vi "GetMeasCatalog.vi"(8 "error in (no error)":errorcluster, 10 "Channel":u32=1, 11 "NetA_AgNA in":refnum<class "NetA_AgNA.lvclass">) -> (0 "error out":errorcluster, 2 "Measurement Catalog":string, 3 "NetA_AgNA out":refnum<class "NetA_AgNA.lvclass">)   [LabVIEW 2014, in "NetA_AgNA.lvclass"]
doc: "Returns a list of measurements associated with the specified channel."
uses:
  NetA_AgNA.lvclass
  NetA_AgNA.lvclass/NetA_AgNA.ctl
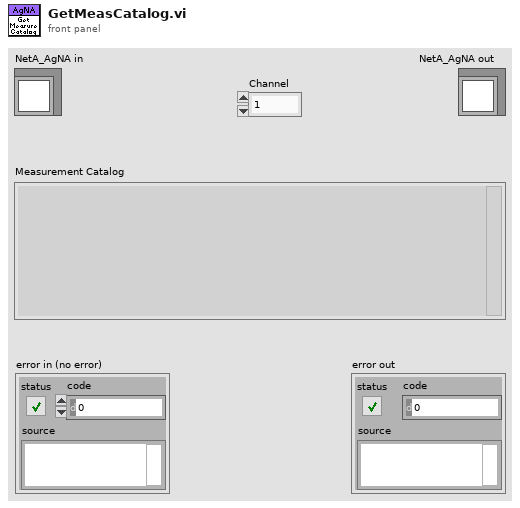
[diagram p1: front panel]
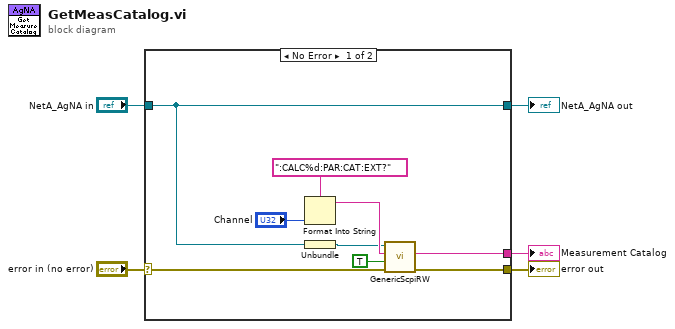
[diagram p0: block diagram]
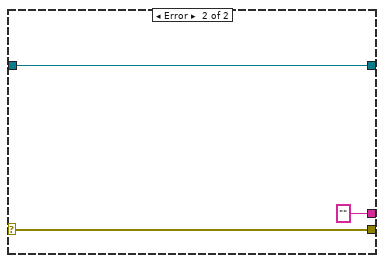
[diagram p2: hidden frame]
diagram:
  n1 = case shown="No Error" "error in (no error)" {
    selector: "error in (no error)" -> [w13 w16]
    tunnel: [w14 w16] -> w5
    tunnel: [w9 "" ("SCPI Response")] -> w3
    tunnel: "NetA_AgNA in" -> [w7 w17]
    tunnel: [w7 w17] -> w1
    frame No Error {
      n2 = Format Into String(format string=":CALC%d:PAR:CAT:EXT?" ("Channel"), "Channel") -> (resulting string=w12:string)  [unwired: 2 in, 1 out]
      n3 = Unbundle(w7) -> (w6:refnum<k15>)
      n4 = call "GenericScpiRW.vi"("error in (no error)"=w13, "Query?"=TRUE, "SCPI Command"=w12, "resource name"=w6) -> ("error out"=w14:errorcluster, "SCPI Response"=w9:string)  [unwired: 6 in]
    }
    frame Error {
    }
  }
  "error out" <- w5
  "Measurement Catalog" <- w3
  "NetA_AgNA out" <- w1
